vi "AC Voltage Configuration.vi"(8 "error in (no error)":errorcluster, 10 "Voltage Range":T1=enum."Auto", 11 "VISA resource name":refnum<visa-resource-name>) -> (0 "error out":errorcluster, 3 "VISA resource name out":refnum<visa-resource-name>)   [LabVIEW 2015, in "Keysight U1252.lvlib"]
uses:
  <instrlib>/Keysight U1252/Keysight U1252.lvlib
  <instrlib>/Keysight U1252/Controls/Voltage Range.ctl
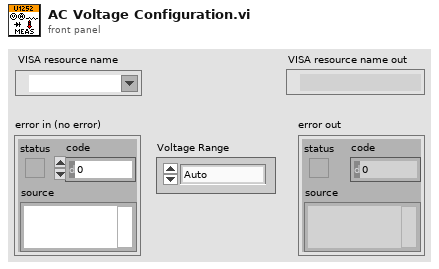
[diagram p1: front panel]
types:
  T1 = typedef "Keysight U1252.lvlib/Voltage Range.ctl" = enum16{"5V", "50V", "500V", "1000V", "Auto"}
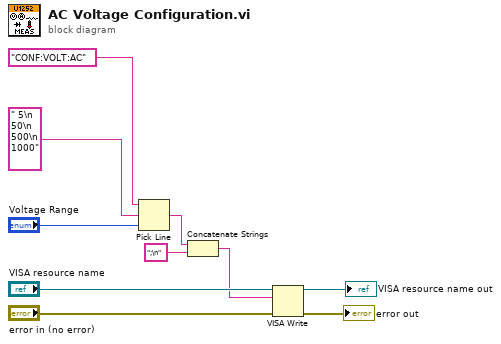
[diagram p0: block diagram]
diagram:
  n1 = Pick Line(string ("")="CONF:VOLT:AC", multi-line string=" 5\n 50\n 500\n 1000", line index="Voltage Range") -> (output string=w3:string)
  n2 = Concatenate Strings(w3, ";\n" ("string")) -> (w1:string)
  n3 = VISA Write(VISA resource name="VISA resource name", write buffer=w1, error in (no error)="error in (no error)") -> (VISA resource name out=→"VISA resource name out":refnum<visa-resource-name>, error out=→"error out":errorcluster)  [unwired: 1 out]
